vi "Test_SetUninstall.vi"(2 "error in":errorcluster, 3 "TestModel":T1, 4 "Uninstall":bool[](array[boolean]), 5 "Contactor":refnum<k21>) -> (0 "error out":errorcluster)   [LabVIEW 2015]
uses:
  CustomControl/Model.ctl
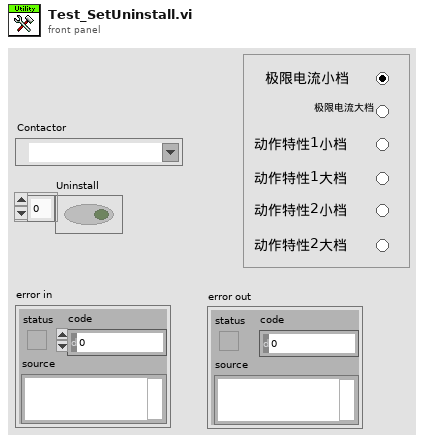
[diagram p1: front panel]
types:
  T1 = typedef "Model.ctl" = enum32{"lowLimit", "upLimit", "lowAction1", "upAction1", "lowAction2", "upAction2"}
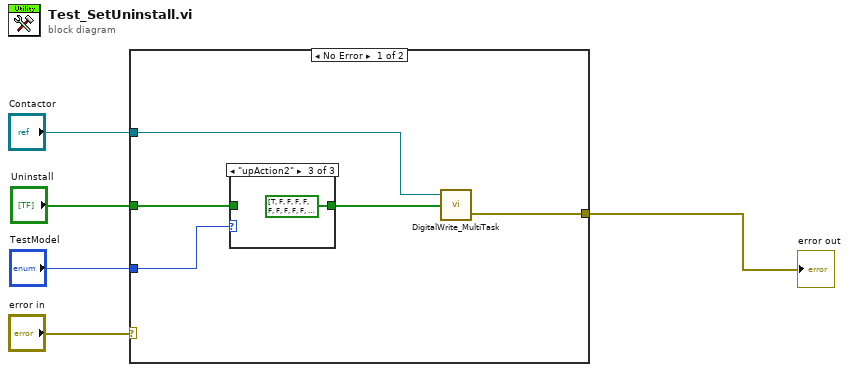
[diagram p0: block diagram]
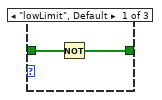
[diagram p2: hidden frame]
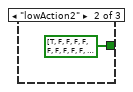
[diagram p3: hidden frame]
diagram:
  n1 = case shown="No Error" "error in" {
    selector: "error in" -> [_ w15]
    tunnel: "Uninstall" -> [w9 _]
    tunnel: "TestModel" -> [w8 _]
    tunnel: [w7 w15] -> w3
    tunnel: "Contactor" -> [w6 _]
    frame No Error {
      n2 = case shown="\"upAction2\"" w8 {
        tunnel: w9 -> [w12 _ _]
        tunnel: [w11 bool[] [TRUE, FALSE, FALSE, FALSE, FALSE, FALSE, FALSE, FALSE, FALSE, FALSE, FALSE, FALSE, FALSE, FALSE, FALSE, FALSE, FALSE, FALSE, FALSE, TRUE] bool[] [TRUE, FALSE, FALSE, FALSE, FALSE, FALSE, FALSE, FALSE, FALSE, FALSE, FALSE, FALSE, FALSE, FALSE, FALSE, FALSE, FALSE, FALSE, FALSE, TRUE]] -> w10
        frame "lowLimit", Default {
          n3 = Not(x=w12) -> (.not. x?=w11:bool[])
        }
        frame "lowAction2" {
        }
        frame "upAction2" {
        }
      }
      n4 = call "DigitalWrite_MultiTask.vi"("input"=w10, "mutiTask"=w6) -> ("error out"=w7:errorcluster)  [unwired: 2 in]
    }
    frame Error {
    }
  }
  "error out" <- w3
